vi "GUIAS CURVAS EM FUNÇÃO DO RAIO-5.vi"() -> ()   [LabVIEW 2014]
uses:
  <vilib>/Platform/TimedLoop/XDataNode/timing_clust.ctl
  <vilib>/Platform/TimedLoop/XDataNode/nitl_modes.ctl
  <vilib>/Platform/TimedLoop/XDataNode/wakeup.ctl
  <vilib>/Platform/TimedLoop/XDataNode/XDataNode.xnode
  <userlib>/Newport ESP301/Newport ESP301.lvlib
  <vilib>/Platform/TimedLoop/XDataNode/XDNodeRunTimeDep.lvlib
  <vilib>/Instr/_visa.llb/VISA Configure Serial Port (Instr).vi
panel:
  out "output cluster 2":T1
  out "output cluster":T1
  in  "Velocity":dbl=3.0
  out "Yin":dbl format="%.6g"
  out "Xin":dbl format="%.6g"
  out "Raio":dbl
  out "PROGRESSÃO":i32
  in  "Raios":dbl[](array[numeric])=[100.0]
  in  "N_Guias":dbl=1.0
  in  "Iniciar":bool
  out "sin(x)":dbl
  in  "L":dbl=10.0 format="%.1f"
  in  "In.Curva":dbl=2.0
  out "d (um)":dbl
  in  "dist.":dbl=100.0
  in  "Stop Button":bool
  out "error out":T3
  out "X (mm)":dbl format="%.2g"
  out "Y (um)":dbl format="%.1f"
  out "XY Graph":cluster{dbl[], dbl[]}(graph)={[0.0, 0.0, 0.0, 0.0, 0.0, 0.0, 0.0, 0.0, 0.0, 0.0, 0.0, 0.0, 0.0, 0.0, 0.0, 0.0, 0.0, 0.0, 0.0, 0.0, 0.0, 0.0, 0.0, 0.0, 0.0, 0.0, 0.0, 0.0, 0.0, 0.0, 0.0, 0.0, 0.0, 0.0, 0.0, 0.0, 0.0, 0.0, 0.0, 0.0, 0.0, 0.0, 0.0, 0.0, 0.0, 0.0, 0.0, 0.0, 0.0, 0.0, 0.0, 0.0, 0.0, 0.0, 0.0, 0.0, 0.0, 0.0, 0.0, 0.0, 0.0, 0.0, 0.0, 0.0, 0.0, 0.0, 0.0, 0.0, 0.0, 0.0, 0.0, 0.0, 0.0, 0.0, 0.0, 0.0], [4600.0, 4600.0, 4600.0, 4600.0, 4600.0, 4600.0, 4600.0, 4600.0, 4600.0, 4600.0, 4600.0, 4600.0, 4600.0, 4600.0, 4600.0, 4600.0, 4600.0, 4600.0, 4600.0, 4600.0, 4600.0, 4600.0, 4600.0, 4600.0, 4600.0, 4600.0, 4600.0, 4690.0, 4802.5, 4800.5, 4799.5, 4799.5, 4799.5, 4800.0, 4800.0, 4800.0, 4800.0, 4800.0, 4800.0, 4800.0, 4800.0, 4800.0, 4800.0, 4800.0, 4995.5, 5001.5, 5000.5, 5000.0, 5000.0, 4999.5, 4999.5, 5000.0, 5000.0, 5000.0, 5000.0, 5000.0, 5000.0, 5000.0, 5000.0, 5000.0, 5000.0, 5000.0, 5000.0, 5000.0, 5000.0, 5000.0, 5000.0, 5000.0, 5000.0, 5000.0, 5000.0, 5000.0, 5000.0, 5000.0, 5000.0, 5000.0]}
  in  "Refresh Button":bool
  # "Inicio curva"
  # "Tamanho da amostra (mm)"
  # "Número guias curvas"
  # "Raio (mm)"
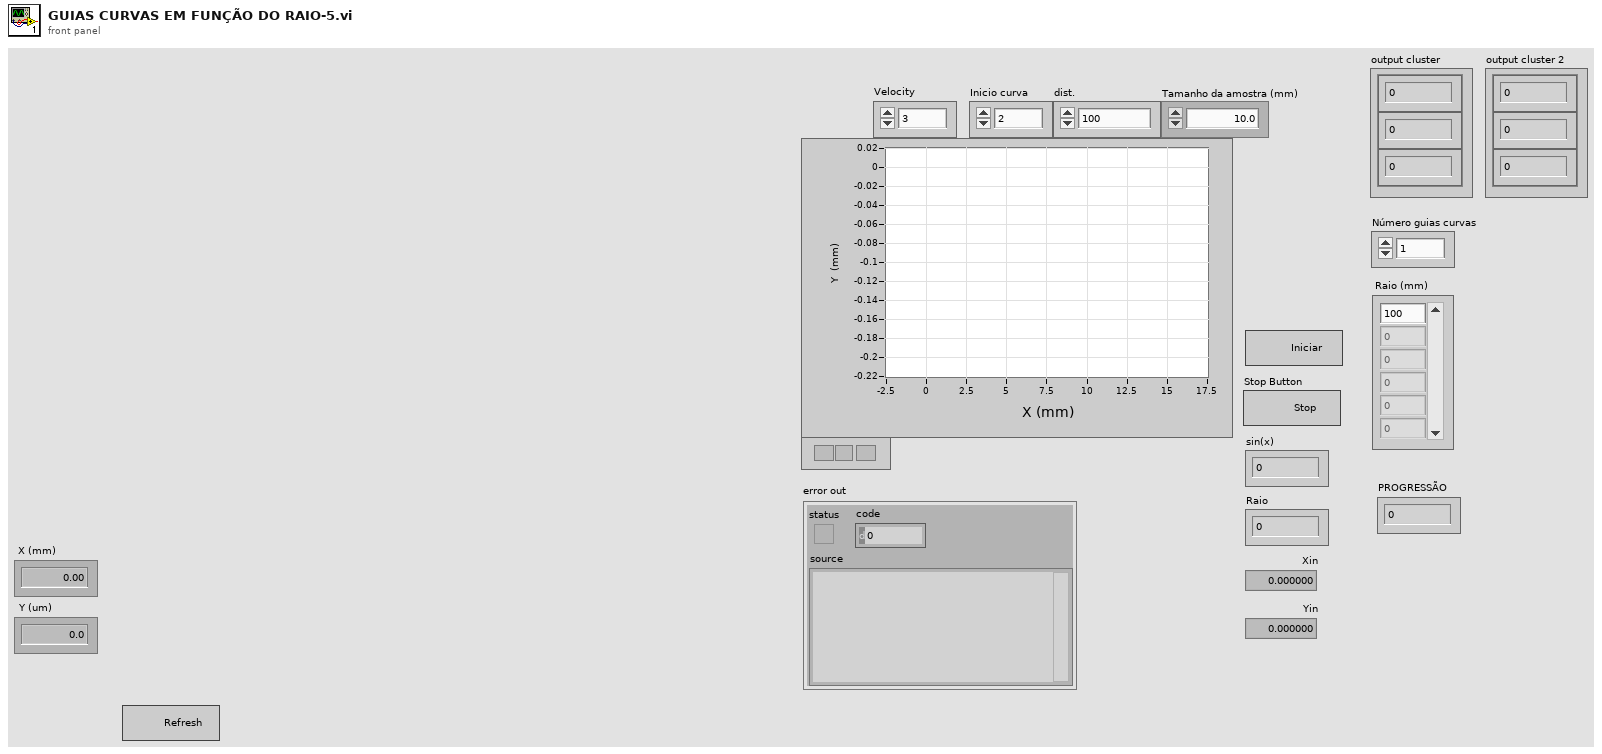
[diagram p1: front panel]
types:
  T1 = cluster{"Numeric Control":dbl, "Numeric Control":dbl, "Numeric Control":dbl}
  T2 = typedef "GUIAS CURVAS EM FUN敲O DO RAIO-6.vi" = bool
  T3 = cluster{"status":T2, "code":i32, "source":string}
  T4 = typedef "XDNodeRunTimeDep.lvlib/timing_clust.ctl" = cluster{"Expected End [f-1]":u64, "Actual End [f-1]":u64, "Finished Late? [f-1]":bool, "Expected End [i-1]":u64, "Actual End [i-1]":u64, "Finished Late? [i-1]":bool, "Expected Start [i]":u64, "Actual Start [i]":u64, "Expected Start [f]":u64, "Actual Start [f]":u64, "Source Name":string, "Structure Name":string, "Period":i64, "Deadline":i64, "Offset":i64, "Start":i64, "Priority":i32, "Timeout":i32, "Mode":T5, "Wakeup Reason":T6, "Error":errorcluster, "Source Type":string, "Secondary Source Type":string, "Global End Time":u64, "Global Start Time":u64, "Frame Duration":u64, "Iteration Duration":u64, "Assigned CPU":i32, "I/O Scan Engine Mode":u32}
  T5 = typedef "XDNodeRunTimeDep.lvlib/nitl_modes.ctl" = enum32{"No Change", "Process missed periods, maintain original phase", "Discard missed periods, maintain original phase", "Process missed periods, ignore original phase", "Discard missed periods, ignore original phase"}
  T6 = typedef "XDNodeRunTimeDep.lvlib/wakeup.ctl" = enum32{"Normal", "Aborted", "Asynchronous wakeup", "Timing source error", "Timed loop error", "Timeout"}
  T7 = cluster{"Axis1 moving":bool, "Axis2 moving":bool, "Axis3 moving":bool, "Axis4 moving":bool, "Motor Power of at least one axis":bool, "Reserved":bool, "Reserved":bool, "Reserved":bool, "Axis5 moving 2":bool, "Axis6 moving 2":bool, "Reserved":bool, "Reserved":bool, "Motor Power of at least one axis":bool, "Reserved":bool, "Reserved":bool, "Reserved":bool}
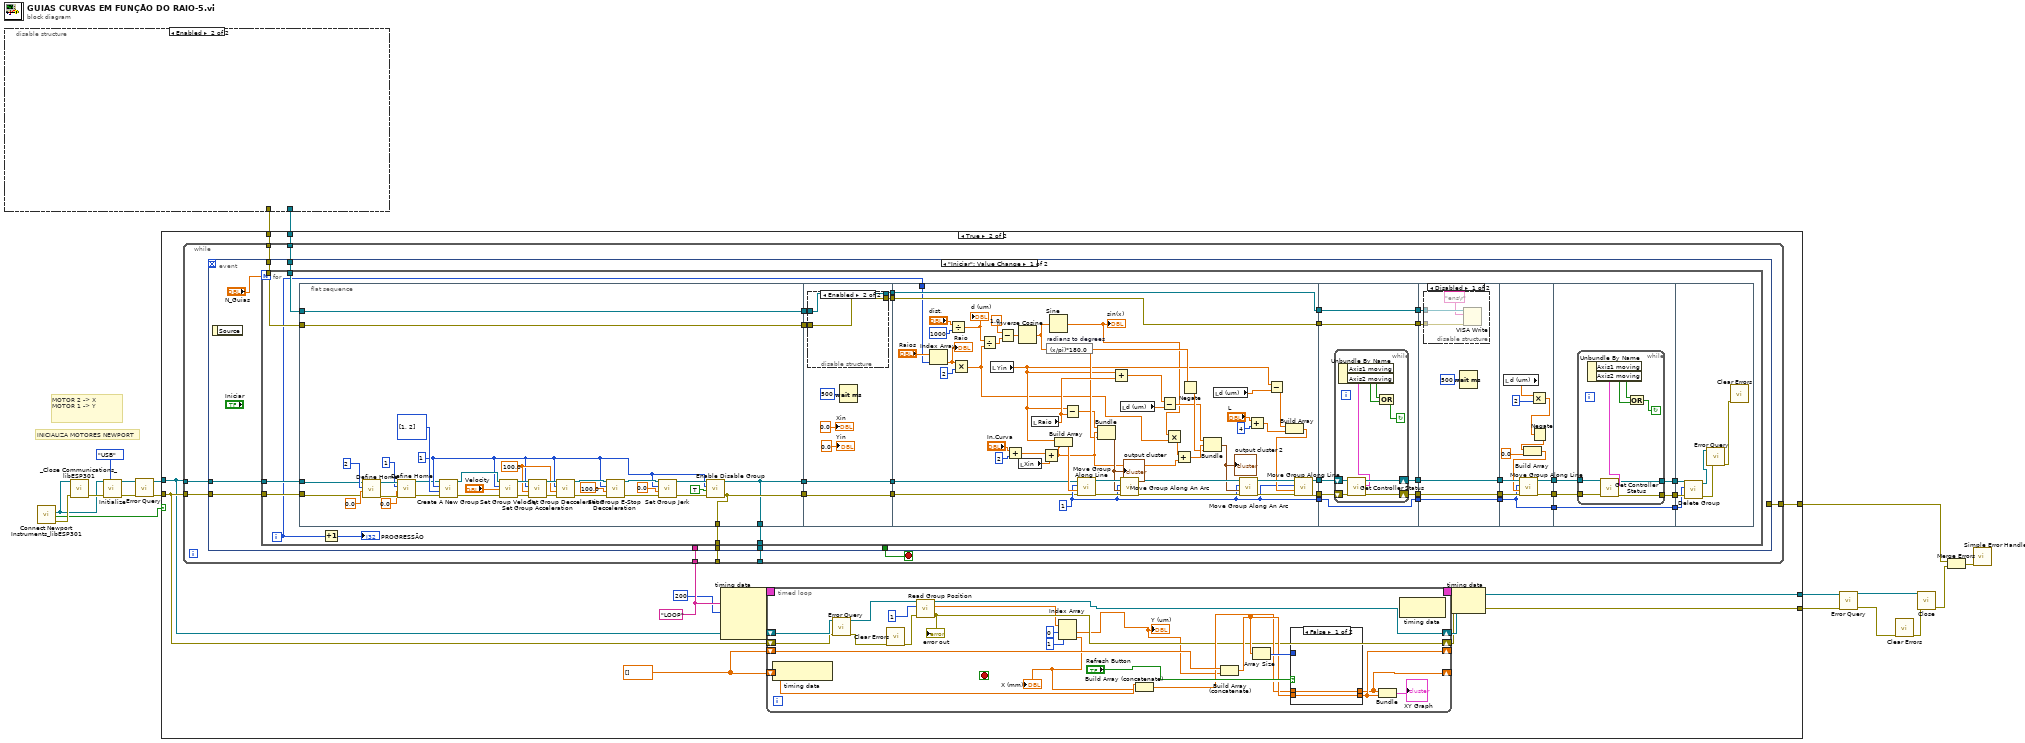
[diagram p0: block diagram]
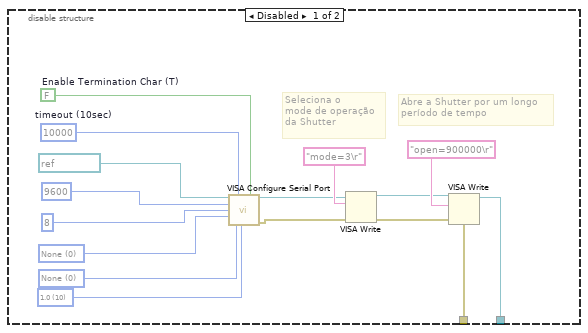
[diagram p2: hidden frame]
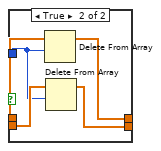
[diagram p4: hidden frame]
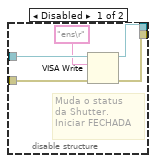
[diagram p5: hidden frame]
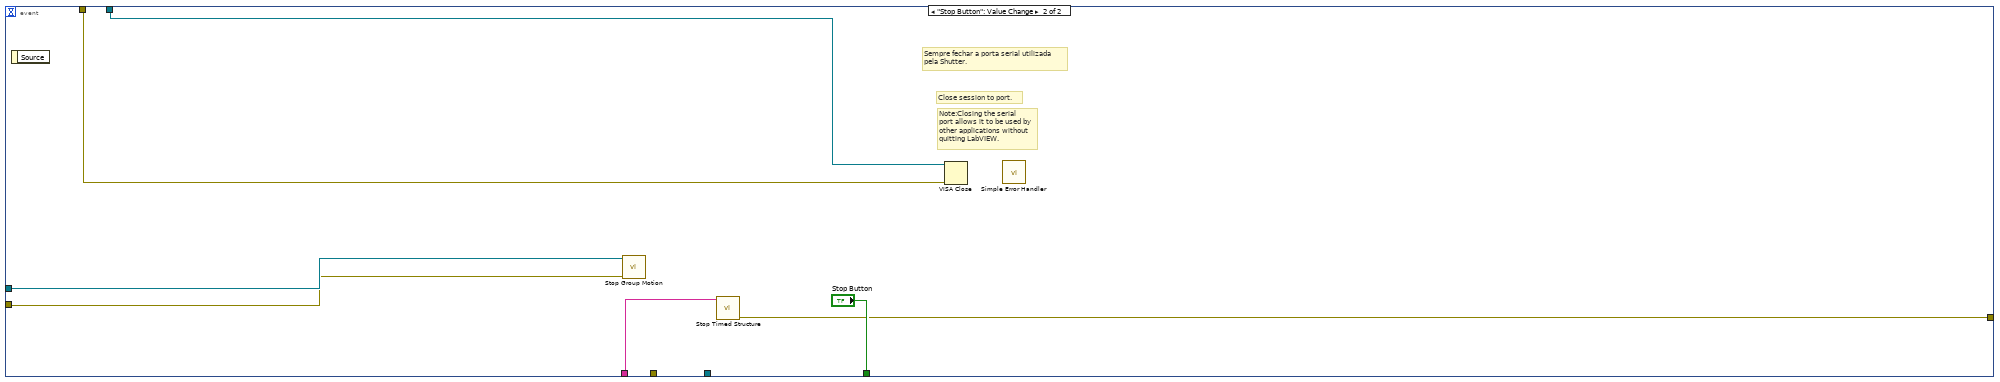
[diagram p7: hidden frame]
diagram:
  # "MOTOR 2 -> X\nMOTOR 1 -> Y"
  # "INICIALIZA MOTORES NEWPORT"
  n1 = disable-structure shown="Enabled" {
    disable-tunnel: [w35 _] -> w7
    disable-tunnel: [w34 _] -> w5
    frame Disabled {
      w28 = u16 0 items=["None", "Odd", "Even", "Mark", "Space"] ("parity")
      w31 = u16 10 items=["1.0"=10, "1.5"=15, "2.0"=20] ("stop bits")
      w32 = u16 0 items=["None"=0, "XON/XOFF"=1, "RTS/CTS"=2, "DTR/DSR"=4] ("flow control")
      w30 = FALSE  # Enable Termination Char (T)
      w29 = u32 10000  # timeout (10sec)
      # "Abre a Shutter por um longo\nperíodo de tempo"
      # "Seleciona o \nmode de operação\nda Shutter"
      n2 = call-poly "VISA Configure Serial Port"("VISA resource name"=refnum<visa-resource-name> "COM6", "timeout (10sec)"=w29, "Enable Termination\nChar (T)"=w30, "baud rate (9600)"=u32 9600 ("baud rate"), "data bits (8)"=u16 8 ("data bits"), "parity (0:none)"=w28, "stop bits (10: 1 bit)"=w31, "flow control (0:none)"=w32) -> ("VISA resource name out"=w24:refnum<visa-resource-name>, "error out"=w23:errorcluster)  [unwired: 6 in]
      n3 = VISA Write(VISA resource name=w24, write buffer="mode=3\r", error in (no error)=w23) -> (VISA resource name out=w21:refnum<visa-resource-name>, error out=w20:errorcluster)  [unwired: 1 out]
      n4 = VISA Write(VISA resource name=w21, write buffer="open=900000\r", error in (no error)=w20) -> (VISA resource name out=w35:refnum<visa-resource-name>, error out=w34:errorcluster)  [unwired: 1 out]
    }
    frame Enabled {
    }
  }
  n5 = call <userlib>:"Connect Newport Instruments_libESP301.vi"() -> ("error (duplicate)"=w17:errorcluster, "Connected"=w6:bool, "VISA resource name (duplicate)"=w16:refnum<visa-resource-name>)  [unwired: 7 in, 2 out]
  n6 = call <userlib>:"_Close Communications_libESP301.vi"("Instrument Channel"=w16, "error in (no error)"=w17) -> ("error out"=w19:errorcluster)  [unwired: 13 in]
  n7 = call <userlib>:"Initialize.vi"("VISA resource name"=w16, "error in (no error)"=w19, "Serial Link (RS232)"=enum16{"RS232", "USB"}."USB") -> ("VISA resource name out"=w15:refnum<visa-resource-name>, "error out"=w14:errorcluster)  [unwired: 6 in]
  n8 = call <userlib>:"Error Query.vi"("error in (no error)"=w14, "VISA resource name"=w15) -> ("error out"=w3:errorcluster, "VISA resource name out"=w4:refnum<visa-resource-name>)  [unwired: 2 in, 2 out]
  n9 = case shown="True" w6 {
    tunnel: [w37 w49] -> w2
    tunnel: [w36 w48] -> w1
    tunnel: w4 -> [w37 w38]
    tunnel: w3 -> [w36 w39]
    tunnel: [_ w46] -> w10
    tunnel: w7 -> [_ w45]
    tunnel: w5 -> [_ w44]
    frame False {
    }
    frame True {
      w40 = dbl[] []
      w47 = "LOOP" ("Structure Name")
      n10 = while {
        tunnel: w39 -> [w94]
        tunnel: w38 -> [w93]
        tunnel: w47 -> [w91]
        tunnel: [w90] -> w46
        tunnel: w45 -> [w89]
        tunnel: w44 -> [w88]
        tunnel: [w87] -> _
        tunnel: [w86] -> _
        stop <- w92 stop-if-true
        n11 = event shown="[0] \"Iniciar\": Value Change" {
          selector: _ -> [_ _]
          dyn-events: _ -> [_ _]
          timeout: _ -> [_ _]
          tunnel: w94 -> [w101 w291]
          tunnel: w93 -> [w100 w292]
          tunnel: [_ "Stop Button"] -> w92
          tunnel: w91 -> [_ w295]
          tunnel: [_ w294] -> w90
          tunnel: w89 -> [w98 w293]
          tunnel: w88 -> [w97 w290]
          tunnel: [w96 _] -> w87
          tunnel: [w95 _] -> w86
          event "Iniciar": Value Change {
            n12 = event-data() -> ()  [unwired: 1 in, 1 out]
            n13 = for {
              N: "N_Guias" -> [_]
              tunnel: w101 -> [w134]
              tunnel: w100 -> [w133]
              tunnel: w98 -> [w131]
              tunnel: w97 -> [w113]
              tunnel: [w103] -> w96
              tunnel: [w102] -> w95
              i -> [w112]
              n14 = flat-sequence {
                tunnel: w113 -> [w168]
                tunnel: w131 -> [w169]
                tunnel: w133 -> [w140]
                tunnel: w134 -> [w139]
                tunnel: [w138] -> w111
                tunnel: [w137] -> w110
                tunnel: [w169] -> w109
                tunnel: [w168] -> w108
                tunnel: [w138] -> w103
                tunnel: [w137] -> w102
                tunnel: [w172] -> w136
                tunnel: [w173] -> w135
                tunnel: [w176] -> w121
                tunnel: [w175] -> w118
                tunnel: w111 -> [w172]
                tunnel: w110 -> [w173]
                tunnel: w109 -> [w177]
                tunnel: w108 -> [w174]
                tunnel: w136 -> [w188]
                tunnel: w135 -> [w189]
                tunnel: w112 -> [w197]
                tunnel: [w202] -> w128
                tunnel: [w201] -> w127
                tunnel: [w200] -> w124
                tunnel: w121 -> [w198]
                tunnel: [w199] -> w119
                tunnel: w118 -> [w199]
                tunnel: [w198] -> w117
                tunnel: [w242] -> w129
                tunnel: w128 -> [w242]
                tunnel: w127 -> [w238]
                tunnel: [w236] -> w126
                tunnel: w124 -> [w239]
                tunnel: [w237] -> w123
                tunnel: [w241] -> w120
                tunnel: w119 -> [w241]
                tunnel: w117 -> [w240]
                tunnel: [w240] -> w116
                tunnel: [w256] -> w130
                tunnel: w129 -> [w256]
                tunnel: w126 -> [w255]
                tunnel: [w255] -> w125
                tunnel: w123 -> [w254]
                tunnel: [w254] -> w122
                tunnel: w120 -> [w253]
                tunnel: w116 -> [w252]
                tunnel: w130 -> [w260]
                tunnel: w125 -> [w270]
                tunnel: w122 -> [w269]
                tunnel: [w263] -> w115
                tunnel: [w262] -> w114
                tunnel: [w260] -> w104
                tunnel: w115 -> [w275]
                tunnel: w114 -> [w274]
                tunnel: [w273] -> w107
                tunnel: [w272] -> w106
                tunnel: [w271] -> w105
                tunnel: w104 -> [w271]
                tunnel: w107 -> [w289]
                tunnel: w106 -> [w288]
                tunnel: w105 -> [w287]
                frame #0 {
                  w149 = 1 ("Group #")
                  w159 = 100.0 ("Acceleration (0 units/s²)")
                  n15 = call <userlib>:"Define Home.vi"("error in (no error)"=w139, "Home Position (0 units)"=0.0, "Axis (1)"=2 ("y"), "VISA resource name"=w140) -> ("error out"=w147:errorcluster, "VISA resource name out"=w148:refnum<visa-resource-name>)  [unwired: 2 in]
                  n16 = call <userlib>:"Define Home.vi"("error in (no error)"=w147, "Home Position (0 units)"=0.0, "Axis (1)"=1, "VISA resource name"=w148) -> ("error out"=w141:errorcluster, "VISA resource name out"=w142:refnum<visa-resource-name>)  [unwired: 2 in]
                  n17 = call <userlib>:"Create A New Group.vi"("error in (no error)"=w141, "Axis Number"=i32[] [1, 2], "Group Number (1)"=w149, "VISA resource name"=w142) -> ("error out"=w165:errorcluster, "VISA resource name out"=w166:refnum<visa-resource-name>)  [unwired: 2 in]
                  n18 = call <userlib>:"Set Group Velocity.vi"("error in (no error)"=w165, "Velocity (units/s)"="Velocity", "Group Number (1)"=w149, "VISA resource name"=w166) -> ("error out"=w160:errorcluster, "VISA resource name out"=w163:refnum<visa-resource-name>)  [unwired: 2 in]
                  n19 = call <userlib>:"Set Group Acceleration.vi"("error in (no error)"=w160, "Acceleration (0 units/s²)"=w159, "Group Number (1)"=w149, "VISA resource name"=w163) -> ("error out"=w161:errorcluster, "VISA resource name out"=w162:refnum<visa-resource-name>)  [unwired: 2 in]
                  n20 = call <userlib>:"Set Group Decceleration.vi"("error in (no error)"=w161, "Decceleration (0 units/s²)"=w159, "Group Number (1)"=w149, "VISA resource name"=w162) -> ("error out"=w155:errorcluster, "VISA resource name out"=w158:refnum<visa-resource-name>)  [unwired: 2 in]
                  n21 = call <userlib>:"Set Group E-Stop Decceleration.vi"("error in (no error)"=w155, "E-Stop Decceleration (0 units/s²)"=100.0, "Group Number (1)"=w149, "VISA resource name"=w158) -> ("error out"=w154:errorcluster, "VISA resource name out"=w157:refnum<visa-resource-name>)  [unwired: 2 in]
                  n22 = call <userlib>:"Set Group Jerk.vi"("error in (no error)"=w154, "Vector Jerk (0 units/s^3)"=0.0, "Group Number (1)"=w149, "VISA resource name"=w157) -> ("error out"=w153:errorcluster, "VISA resource name out"=w156:refnum<visa-resource-name>)  [unwired: 2 in]
                  n23 = call <userlib>:"Enable Disable Group.vi"("error in (no error)"=w153, "Action (OFF)"=TRUE, "Group Number (1)"=w149, "VISA resource name"=w156) -> ("error out"=w138:errorcluster, "VISA resource name out"=w137:refnum<visa-resource-name>)  [unwired: 2 in]
                }
                frame #1 {
                  n24 = disable-structure shown="Enabled" {
                    disable-tunnel: w177 -> [w183 w185]
                    disable-tunnel: [w182 w185] -> w176
                    disable-tunnel: [w181 w184] -> w175
                    disable-tunnel: w174 -> [w180 w184]
                    frame Disabled {
                      # "Muda o status\nda Shutter.\nIniciar FECHADA"
                      n25 = VISA Write(VISA resource name=w183, write buffer="ens\r", error in (no error)=w180) -> (VISA resource name out=w182:refnum<visa-resource-name>, error out=w181:errorcluster)  [unwired: 1 out]
                    }
                    frame Enabled {
                    }
                  }
                  n26 = Wait (ms)(milliseconds to wait=u32 500) -> ()  [unwired: 1 out]
                  "Xin" <- 0.0 ("Xin")
                  "Yin" <- 0.0 ("Yin")
                }
                frame #2 {
                  w202 = 1 ("y")
                  n27 = Index Array(array="Raios", index=w197) -> (element=w203:dbl)
                  "Raio" <- w203
                  n28 = Divide(x="dist.", y=1000) -> (x/y=w226:dbl)
                  "d (um)" <- w226
                  n29 = Multiply(x=w203, y=2) -> (x*y=w187:dbl)
                  n30 = Divide(x=w226, y=w187) -> (x/y=w229:dbl)
                  n31 = local read "Yin"() -> (w195:dbl)
                  n32 = Subtract(x=1.0, y=w229) -> (x-y=w227:dbl)
                  n33 = Add(x="In.Curva", y=2) -> (x+y=w215:dbl)
                  n34 = Inverse Cosine(1:w227) -> (0:w216:dbl)
                  n35 = local read "Xin"() -> (w217:dbl)
                  n36 = local read "Raio"() -> (w211:dbl)
                  n37 = Add(x=w215, y=w217) -> (x+y=w213:dbl)
                  n38 = expression code="(x/pi)*180.0" "radians to degrees"(w216) -> (w207:dbl)
                  n39 = Sine(x=w216) -> (sin(x)=w186:dbl)
                  "sin(x)" <- w186
                  n40 = Build Array(w195, w213) -> (w223:dbl[])
                  n41 = Subtract(x=w195, y=w211) -> (x-y=w194:dbl)
                  n42 = call <userlib>:"Move Group Along Line.vi"("error in (no error)"=w188, "Position (0 units)"=w223, "Group Number (1)"=w202, "VISA resource name"=w189) -> ("error out"=w221:errorcluster, "VISA resource name out"=w222:refnum<visa-resource-name>)  [unwired: 2 in]
                  n43 = Bundle(w194, w213, w207) -> (w220:cluster{dbl, dbl, dbl})  [unwired: 1 in]
                  "output cluster" <- w220
                  n44 = Add(x=w195, y=w211) -> (x+y=w191:dbl)
                  n45 = local read "d (um)"() -> (w192:dbl)
                  n46 = call <userlib>:"Move Group Along An Arc.vi"("error in (no error)"=w221, "Arc  Parameters"=w220, "Group Number (1)"=w202, "VISA resource name"=w222) -> ("error out"=w234:errorcluster, "VISA resource name out"=w235:refnum<visa-resource-name>)  [unwired: 2 in]
                  n47 = Subtract(x=w191, y=w192) -> (x-y=w190:dbl)
                  n48 = Multiply(x=w186, y=w187) -> (x*y=w214:dbl)
                  n49 = Add(x=w214, y=w213) -> (x+y=w212:dbl)
                  n50 = Negate(x=w207) -> (-x=w206:dbl)
                  n51 = Bundle(w190, w212, w206) -> (w233:cluster{dbl, dbl, dbl})  [unwired: 1 in]
                  "output cluster 2" <- w233
                  n52 = local read "d (um)"() -> (w193:dbl)
                  n53 = call <userlib>:"Move Group Along An Arc.vi"("error in (no error)"=w234, "Arc  Parameters"=w233, "Group Number (1)"=w202, "VISA resource name"=w235) -> ("error out"=w205:errorcluster, "VISA resource name out"=w210:refnum<visa-resource-name>)  [unwired: 2 in]
                  n54 = Add(x="L", y=4) -> (x+y=w209:dbl)
                  n55 = Subtract(x=w195, y=w193) -> (x-y=w196:dbl)
                  n56 = Build Array(w196, w209) -> (w208:dbl[])
                  n57 = call <userlib>:"Move Group Along Line.vi"("error in (no error)"=w205, "Position (0 units)"=w208, "Group Number (1)"=w202, "VISA resource name"=w210) -> ("error out"=w201:errorcluster, "VISA resource name out"=w200:refnum<visa-resource-name>)  [unwired: 2 in]
                }
                frame #3 {
                  n58 = while {
                    shift-right: [w248] -> w237
                    shift-left: w239 -> [w250]
                    shift-right: [w247] -> w236
                    shift-left: w238 -> [w249]
                    stop <- w243 continue-if-true
                    n59 = call <userlib>:"Get Controller Status.vi"("error in (no error)"=w249, "VISA resource name"=w250) -> ("error out"=w247:errorcluster, "Controller Status"=w246:T7, "VISA resource name out"=w248:refnum<visa-resource-name>)  [unwired: 2 in, 1 out]
                    n60 = Unbundle By Name(w246) -> ("Axis1 moving"=w245:bool, "Axis2 moving"=w244:bool)
                    n61 = Compound Arithmetic op=OR(w245, w244) -> (w243:bool)
                  }
                }
                frame #4 {
                  n62 = disable-structure shown="Disabled" {
                    disable-tunnel: w253 -> [w259 _]
                    disable-tunnel: w252 -> [w258 _]
                    frame Disabled {
                      n63 = VISA Write(VISA resource name=w258, write buffer="ens\r", error in (no error)=w259) -> ()  [unwired: 3 out]
                    }
                    frame Enabled {
                    }
                  }
                  n64 = Wait (ms)(milliseconds to wait=u32 500) -> ()  [unwired: 1 out]
                }
                frame #5 {
                  n65 = local read "d (um)"() -> (w266:dbl)
                  n66 = Multiply(x=w266, y=2) -> (x*y=w261:dbl)
                  n67 = Negate(x=w261) -> (-x=w264:dbl)
                  n68 = Build Array(w264, 0.0 ("element")) -> (w268:dbl[])
                  n69 = call <userlib>:"Move Group Along Line.vi"("error in (no error)"=w270, "Position (0 units)"=w268, "Group Number (1)"=w260, "VISA resource name"=w269) -> ("error out"=w262:errorcluster, "VISA resource name out"=w263:refnum<visa-resource-name>)  [unwired: 2 in]
                }
                frame #6 {
                  n70 = while {
                    tunnel: w275 -> [w279]
                    tunnel: w274 -> [w278]
                    tunnel: [w277] -> w273
                    tunnel: [w276] -> w272
                    stop <- w280 continue-if-true
                    n71 = call <userlib>:"Get Controller Status.vi"("error in (no error)"=w278, "VISA resource name"=w279) -> ("error out"=w276:errorcluster, "Controller Status"=w283:T7, "VISA resource name out"=w277:refnum<visa-resource-name>)  [unwired: 2 in, 1 out]
                    n72 = Unbundle By Name(w283) -> ("Axis1 moving"=w282:bool, "Axis2 moving"=w281:bool)
                    n73 = Compound Arithmetic op=OR(w282, w281) -> (w280:bool)
                  }
                }
                frame #7 {
                  n74 = call <userlib>:"Delete Group.vi"("error in (no error)"=w288, "Group Number (1)"=w287, "VISA resource name"=w289) -> ("error out"=w284:errorcluster, "VISA resource name out"=w285:refnum<visa-resource-name>)  [unwired: 3 in]
                  n75 = call <userlib>:"Error Query.vi"("error in (no error)"=w284, "VISA resource name"=w285) -> ("error out"=w286:errorcluster)  [unwired: 2 in, 3 out]
                  n76 = call <vilib>:"Clear Errors.vi"("error in (no error)"=w286) -> ()  [unwired: 5 in, 2 out]
                }
              }
              n77 = Increment(x=w112) -> (x+1=→"PROGRESSÃO":i32)
            }
          }
          event "Stop Button": Value Change {
            # "Sempre fechar a porta serial utilizada\npela Shutter."
            # "Note:Closing the serial port allows it to be used by other applications without\nquitting LabVIEW."
            # "Close session to port."
            n78 = event-data() -> ()  [unwired: 1 in, 1 out]
            n79 = call <userlib>:"Stop Group Motion.vi"("error in (no error)"=w291, "VISA resource name"=w292) -> ()  [unwired: 4 in, 2 out]
            n80 = call <vilib>:"Stop Timed Structure.vi"("name"=w295) -> ("error out"=w294:errorcluster)  [unwired: 10 in]
            n81 = VISA Close(VISA resource name=w293, error in (no error)=w290) -> ()  [unwired: 1 out]
            n82 = call <vilib>:"Simple Error Handler.vi"() -> ()  [unwired: 5 in, 5 out]
          }
        }
      }
      n83 = node-c288(w47, i64 200 ("Period")) -> (w43:T4)  [unwired: 2 in]
      n84 = timed-loop {
        timing: w43 -> [_]
        timing-out: [_] -> w42
        shift-right: [w61] -> w49
        shift-left: w38 -> [w54]
        shift-right: [w60] -> w48
        shift-left: w39 -> [w53]
        shift-right: [w64] -> _
        shift-left: w40 -> [w68]
        shift-right: [w63] -> _
        shift-left: w40 -> [w66]
        stop <- _ stop-if-true
        n85 = node-c288() -> ()  [unwired: 1 in, 1 out]
        n86 = call <userlib>:"Error Query.vi"("error in (no error)"=w53, "VISA resource name"=w54) -> ("error out"=w51:errorcluster, "VISA resource name out"=w52:refnum<visa-resource-name>)  [unwired: 2 in, 2 out]
        n87 = call <vilib>:"Clear Errors.vi"("error in (no error)"=w51) -> ("error out"=w50:errorcluster)  [unwired: 5 in, 1 out]
        n88 = call <userlib>:"Read Group Position.vi"("error in (no error)"=w50, "Group Number (1)"=1, "VISA resource name"=w52) -> ("error out"=w60:errorcluster, "Position (units)"=w57:dbl[], "VISA resource name out"=w61:refnum<visa-resource-name>)  [unwired: 2 in]
        "error out" <- w60
        n89 = Index Array(array=w57, index #1=0 ("index"), index #2=1 ("index")) -> (element #1=w56:dbl, element #2=w55:dbl)
        "X (mm)" <- w55
        "Y (um)" <- w56
        n90 = Build Array (concatenate)(w66, w55) -> (w65:dbl[])
        n91 = Build Array (concatenate)(w68, w56) -> (w67:dbl[])
        n92 = Array Size(array=w67) -> (size(s)=w69:i32)
        n93 = case shown="False" "Refresh Button" {
          tunnel: [w73 w75] -> w63
          tunnel: w65 -> [w73 w78]
          tunnel: [w72 w74] -> w64
          tunnel: w67 -> [w72 w77]
          tunnel: w69 -> [_ w76]
          frame False {
          }
          frame True {
            n94 = Delete From Array(array=w78, length=w76) -> (array with subset deleted=w75:dbl[])  [unwired: 1 in, 1 out]
            n95 = Delete From Array(array=w77, length=w76) -> (array with subset deleted=w74:dbl[])  [unwired: 1 in, 1 out]
          }
        }
        n96 = Bundle(w63, w64) -> (→"XY Graph":cluster{dbl[], dbl[]})  [unwired: 1 in]
        n97 = node-c288() -> ()  [unwired: 1 in, 1 out]
      }
      n98 = node-c288(w42) -> ()  [unwired: 1 out]
    }
  }
  n99 = call <userlib>:"Error Query.vi"("error in (no error)"=w1, "VISA resource name"=w2) -> ("error out"=w11:errorcluster, "VISA resource name out"=w12:refnum<visa-resource-name>)  [unwired: 2 in, 2 out]
  n100 = call <vilib>:"Clear Errors.vi"("error in (no error)"=w11) -> ("error out"=w13:errorcluster)  [unwired: 5 in, 1 out]
  n101 = call <userlib>:"Close.vi"("error in (no error)"=w13, "VISA resource name"=w12) -> ("error out"=w9:errorcluster)  [unwired: 9 in]
  n102 = Merge Errors(w10, w9) -> (w8:errorcluster)
  n103 = call <vilib>:"Simple Error Handler.vi"("error in (no error)"=w8) -> ()  [unwired: 4 in, 5 out]
